vi "New dotNET WebSocket Client.vi"(7 "Client SSL Options (wss://)":T1={"Check Revocation"=FALSE, "SSL Protocols"=[240], "Client Certs"=[]} {"SSL Protocols" items=["None"=0, "Ssl2"=12, "Ssl3"=48, "Tls"=192, "Default"=240, "Tls11"=768, "Tls12"=3072]}, 8 "error in (no error)":errorcluster, 9 "Timeout (5000ms)":i32=5000, 11 "WebSocket URL":string="wss://localhost:7123") -> (0 "error out":errorcluster, 3 "dotNET WS Client out":refnum<class "dotNET WebSocket Client.lvclass">)   [LabVIEW 2013, in "dotNET WebSocket.lvlib" / "dotNET WebSocket Client.lvclass"]
doc: "Opens a new client connection to the given websockets URL using a dotNET socket. Supports ws:// and wss:// protocols."
uses:
  dotNET WebSocket Client.lvclass
  SSL Client Options.ctl
  dotNET SSL Socket/PFX Certificate.ctl
  dotNET SSL Socket/dotNET SSL Socket.lvclass/dotNET SSL Socket.ctl
  dotNET SSL Client/dotNET SSL Client Socket.lvclass/dotNET SSL Client Socket.ctl
  dotNET SSL Client/dotNET SSL Client Socket.lvclass
  <vilib>/MediaMongrels Ltd/WebSockets/WebSockets/WebSocket/WebSocket.lvclass/WebSocket.ctl
  <vilib>/MediaMongrels Ltd/WebSockets/WebSockets/WebSocket Client/WebSocket Client.lvclass/WebSocket Client.ctl
  dotNET SSL Socket/Write Check Revocation.vi
  dotNET SSL Socket/Write SSL Protocols.vi
  dotNET SSL Client/Write Client Certs.vi
  <vilib>/MediaMongrels Ltd/WebSockets/WebSockets/WebSocket/Write Socket.vi
  <vilib>/MediaMongrels Ltd/WebSockets/WebSockets/WebSocket Client/Write URL.vi
  dotNET TCP Socket/dotNET TCP Socket.lvclass
  <vilib>/MediaMongrels Ltd/WebSockets/WebSockets/WebSocket/WebSocket.lvclass
  <vilib>/MediaMongrels Ltd/WebSockets/WebSockets/WebSocket Client/WebSocket Client.lvclass
  dotNET SSL Socket/dotNET SSL Socket.lvclass
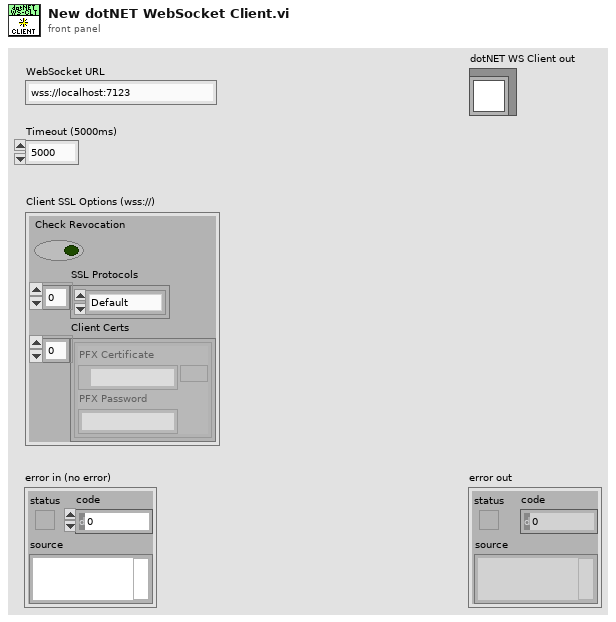
[diagram p1: front panel]
types:
  T1 = typedef "dotNET WebSocket.lvlib/dotNET WebSocket Client.lvclass/SSL Client Options.ctl" = cluster{"Check Revocation":bool, "SSL Protocols":i32[], "Client Certs":T2[]}
  T2 = typedef "dotNET SSL Socket.lvlib/dotNET SSL Socket.lvclass/PFX Certificate.ctl" = cluster{"PFX Certificate":path, "PFX Password":string}
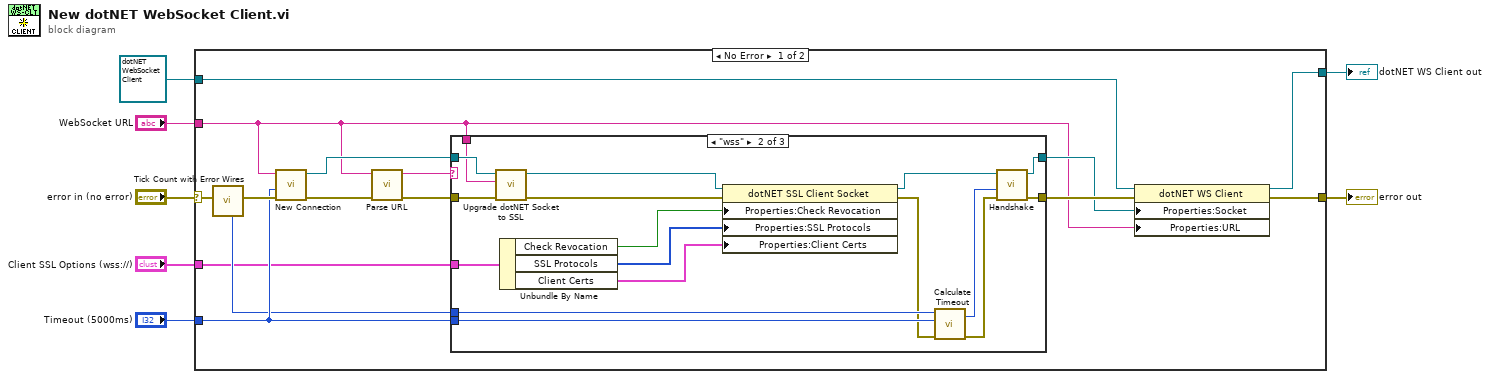
[diagram p0: block diagram]
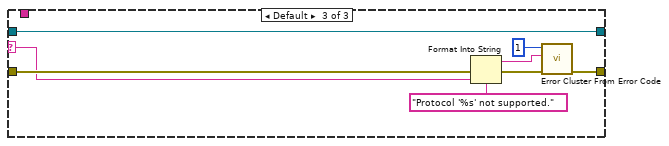
[diagram p3: hidden frame]
diagram:
  n1 = case shown="No Error" "error in (no error)" {
    selector: "error in (no error)" -> [w16 w51]
    tunnel: [w20 w51] -> w6
    tunnel: [w17 w50] -> w3
    tunnel: "WebSocket URL" -> [w10 _]
    tunnel: "Timeout (5000ms)" -> [w14 _]
    tunnel: refnum<class "dotNET WebSocket Client.lvclass"> refnum ("dotNET WS Client out") -> [w19 w50]
    tunnel: "Client SSL Options (wss://)" -> [w8 _]
    frame No Error {
      n2 = call <vilib>:"Tick Count with Error Wires.vi"("error in (no error)"=w16) -> ("error out"=w15:errorcluster, "millisecond timer value"=w13:u32)  [unwired: 9 in]
      n3 = call "New Connection.vi"("error in (no error)"=w15, "Timeout (5000ms)"=w14, "Hostname / URL"=w10) -> ("error out"=w12:errorcluster, "dotNET TCP Socket out"=w22:refnum<class "dotNET TCP Socket.lvclass">)  [unwired: 7 in]
      n4 = call <vilib>:"Parse URL.vi"("error in (no error)"=w12, "WebSocket URL"=w10) -> ("error out"=w11:errorcluster, "protocol"=w9:string)  [unwired: 5 in, 3 out]
      n5 = case shown="\"wss\"" w9 {
        selector: w9 -> [_ _ w43]
        tunnel: w22 -> [w24 w41 w49]
        tunnel: w11 -> [w23 w40 w47]
        tunnel: [w23 w39 w48] -> w21
        tunnel: w10 -> [_ w38 _]
        tunnel: [w24 w37 w49] -> w18
        tunnel: w14 -> [_ w36 _]
        tunnel: w13 -> [_ w35 _]
        tunnel: w8 -> [_ w28 _]
        frame "ws" {
        }
        frame "wss" {
          n6 = call "Upgrade dotNET Socket to SSL.vi"("error in (no error)"=w40, "Hostname / URL"=w38, "dotNET TCP Socket in"=w41) -> ("error out"=w34:errorcluster, "dotNET SSL Client Socket out"=w30:refnum<class "dotNET SSL Client Socket.lvclass">)  [unwired: 7 in]
          n7 = Unbundle By Name(w28) -> ("Check Revocation"=w27:bool, "SSL Protocols"=w26:i32[], "Client Certs"=w25:T2[])
          n8 = property class="dotNET SSL Client Socket"(reference=w30, error in=w34, "Properties:Check Revocation"=w27, "Properties:SSL Protocols"=w26, "Properties:Client Certs"=w25) -> (reference out=w29:refnum<class "dotNET SSL Client Socket.lvclass">, error out=w31:errorcluster)
          n9 = call <vilib>:"Calculate Timeout.vi"("error in (no error)"=w31, "timeout ms"=w36, "t0"=w35) -> ("error out"=w33:errorcluster, "new timeout ms"=w32:i32)  [unwired: 6 in, 1 out]
          n10 = call-dynamic "Handshake.vi"("error in (no error)"=w33, "Timeout (5000ms)"=w32, "dotNET SSL Client Socket in"=w29) -> ("error out"=w39:errorcluster, "dotNET SSL Client Socket out"=w37:refnum<class "dotNET SSL Client Socket.lvclass">)  [unwired: 7 in]
        }
        frame Default {
          n11 = Format Into String(format string="Protocol '%s' not supported.", error in=w47, w43) -> (resulting string=w45:string, error out=w46:errorcluster)  [unwired: 1 in]
          n12 = call <vilib>:"Error Cluster From Error Code.vi"("error in (no error)"=w46, "error message (\"\")"=w45, "error code (0)"=1) -> ("error out"=w48:errorcluster)  [unwired: 6 in]
        }
      }
      n13 = property class="dotNET WS Client"(reference=w19, error in=w21, "Properties:Socket"=w18, "Properties:URL"=w10) -> (reference out=w17:refnum<class "dotNET WebSocket Client.lvclass">, error out=w20:errorcluster)
    }
    frame Error {
    }
  }
  "error out" <- w6
  "dotNET WS Client out" <- w3
